vi "Send Command (non-enum).vi"(8 "error in (no error)":errorcluster, 10 "Commands":string[](array[string]), 11 "Hitronics in":refnum<class "Hitronics.lvclass">) -> (0 "error out":errorcluster, 3 "Hitronics out":refnum<class "Hitronics.lvclass">)   [LabVIEW 2018, in "Hitronics.lvlib" / "Hitronics.lvclass"]
doc: "This Override can send multiple commands that do not require a response from the targeted device."
uses:
  Hitronics.lvclass
  PPLs/Laser/Parent/Laser.lvlibp/Laser.lvclass
  C:/AME Test Engineering/LabVIEW/PPLs/Laser/Parent/Laser.lvlibp/Laser.lvclass
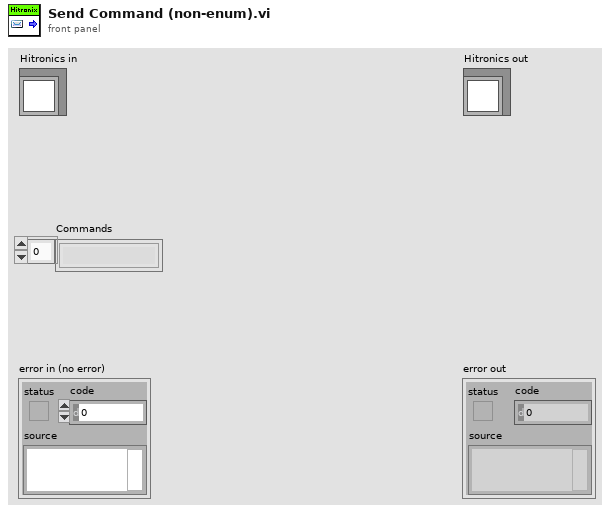
[diagram p1: front panel]
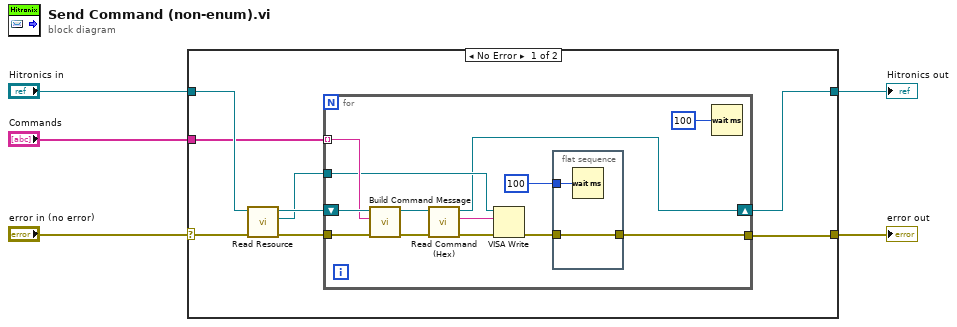
[diagram p0: block diagram]
diagram:
  n1 = case shown="No Error" "error in (no error)" {
    selector: "error in (no error)" -> [w13 w29]
    tunnel: "Hitronics in" -> [w12 w30]
    tunnel: "Commands" -> [w10 _]
    tunnel: [w7 w30] -> w2
    tunnel: [w6 w29] -> w1
    frame No Error {
      n2 = call "Read Resource.vi"("error in (no error)"=w13, "Laser in"=w12) -> ("error out"=w9:errorcluster, "Resource"=w8:refnum<visa-resource-name>, "Laser out"=w11:refnum<class "Hitronics.lvclass">)  [unwired: 7 in]
      n3 = for {
        tunnel: w10 -> [w25] mode=indexing
        tunnel: w9 -> [w24]
        tunnel: w8 -> [w21]
        shift-right: [w15] -> w7
        shift-left: w11 -> [w26]
        tunnel: [w16] -> w6
        n4 = call "Build Command Message.vi"("error in (no error)"=w24, "Command"=w25, "Hitronics in"=w26) -> ("error out"=w22:errorcluster, "Hitronics out"=w23:refnum<class "Hitronics.lvclass">)  [unwired: 7 in]
        n5 = call-dynamic "Read Command (Hex).vi"("error in (no error)"=w22, "Hitronics in"=w23) -> ("error out"=w20:errorcluster, "Command (Hex)"=w14:string, "Hitronics out"=w15:refnum<class "Hitronics.lvclass">)  [unwired: 7 in]
        n6 = VISA Write(VISA resource name=w21, write buffer=w14, error in (no error)=w20) -> (error out=w17:errorcluster)  [unwired: 2 out]
        n7 = flat-sequence {
          tunnel: u32 100 ("milliseconds to wait") -> [w28]
          tunnel: w17 -> [w27]
          tunnel: [w27] -> w16
          frame #0 {
            n8 = Wait (ms)(milliseconds to wait=w28) -> ()  [unwired: 1 out]
          }
        }
        n9 = Wait (ms)(milliseconds to wait=u32 100) -> ()  [unwired: 1 out]
      }
    }
    frame Error {
    }
  }
  "error out" <- w1
  "Hitronics out" <- w2
